vi "Parse Value.vi"(8 "error in (no error)":errorcluster, 11 "Alpaca CLI Parser in":refnum<class "JSON Parser.lvclass">) -> (0 "error out":errorcluster, 2 "Value":variant, 3 "Alpaca CLI Parser out":refnum<class "JSON Parser.lvclass">)   [LabVIEW 2013, in "JKI JSON Serialization.lvlib" / "JSON Parser.lvclass"]
uses:
  JSON Parser.lvclass
  Parser/Parser.lvclass/Parser.ctl
  JSON Lexer/JSON Token Type.ctl
  Parser/Lookahead.vi
  JSON Lexer/JSON Lexer.lvclass
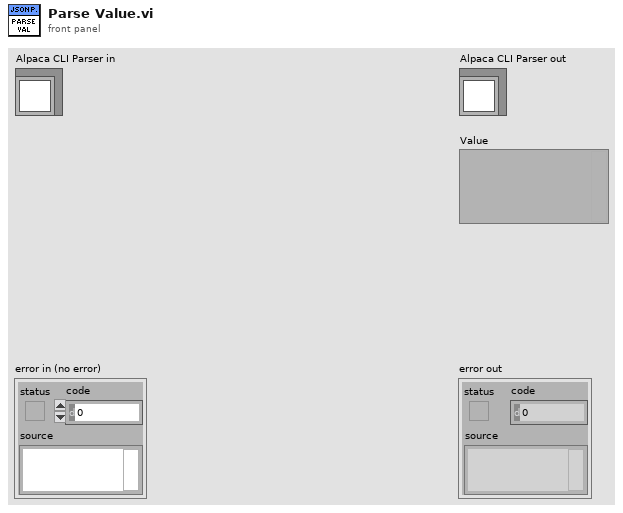
[diagram p1: front panel]
types:
  T1 = typedef "JKI JSON Serialization.lvlib/JSON Lexer.lvclass/JSON Token Type.ctl" = enum32{"unknown", "comma", "end-label", "begin-object", "end-object", "begin-array", "end-array", "quoted-string", "boolean", "exponential-number", "decimal-number", "integer-number", "special-number", "null", "symbol", "whitespace", "EOF"}
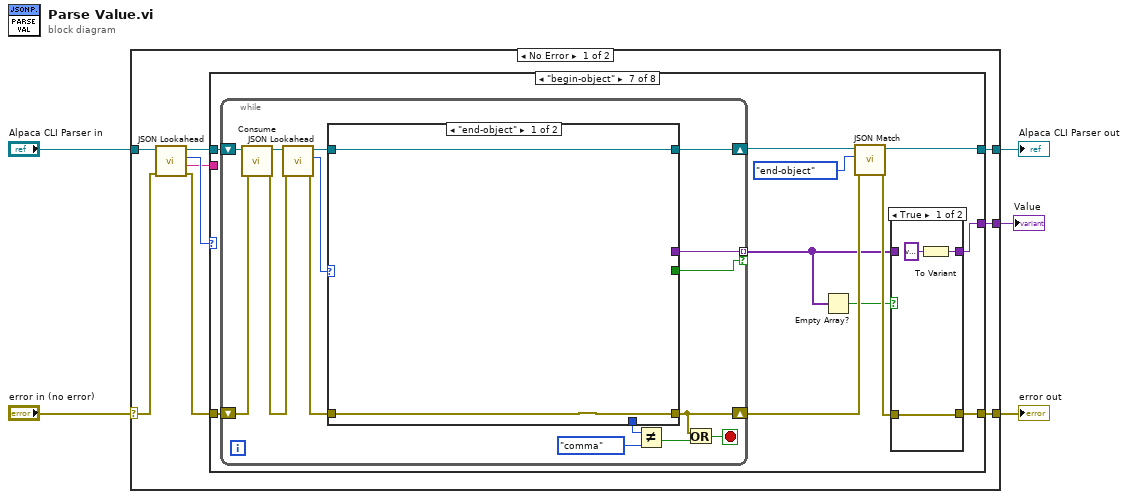
[diagram p0: block diagram]
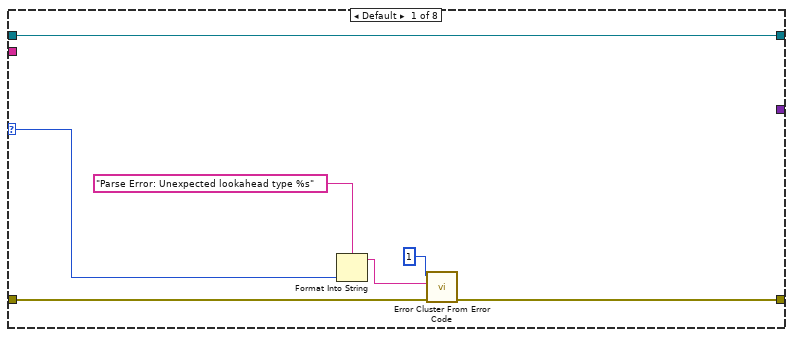
[diagram p2: hidden frame]
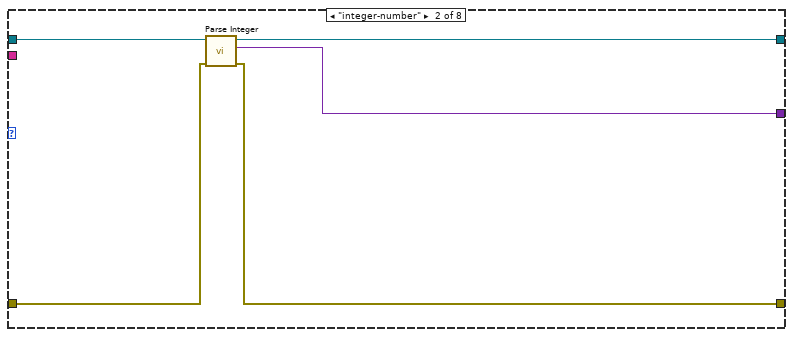
[diagram p3: hidden frame]
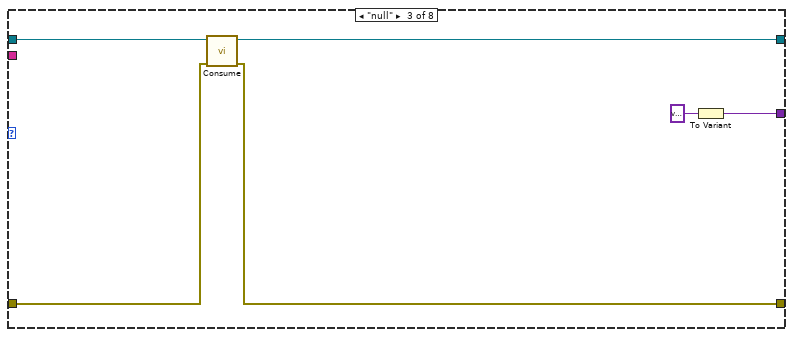
[diagram p4: hidden frame]
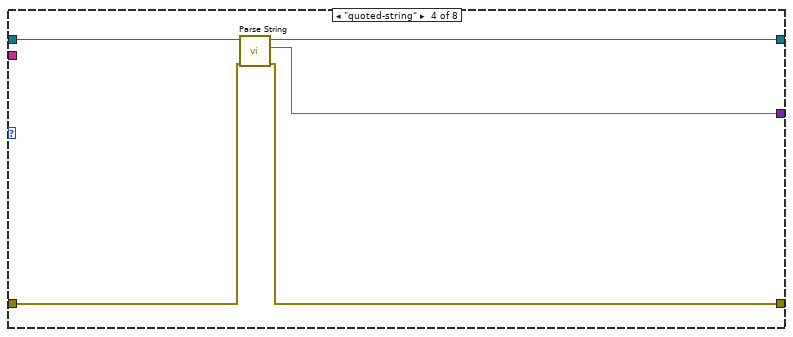
[diagram p5: hidden frame]
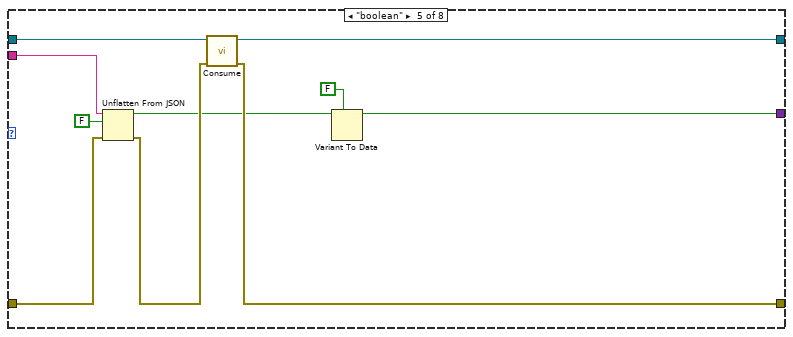
[diagram p6: hidden frame]
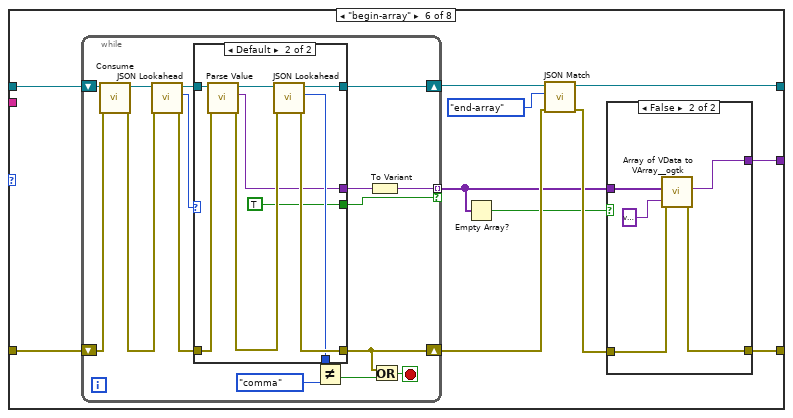
[diagram p7: hidden frame]
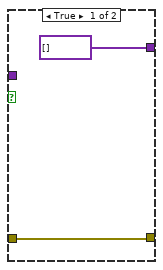
[diagram p8: hidden frame]
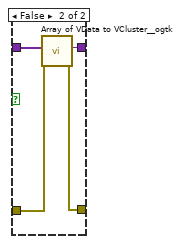
[diagram p10: hidden frame]
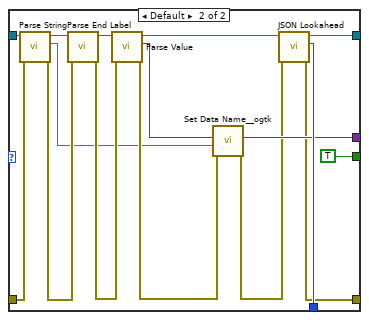
[diagram p11: hidden frame]
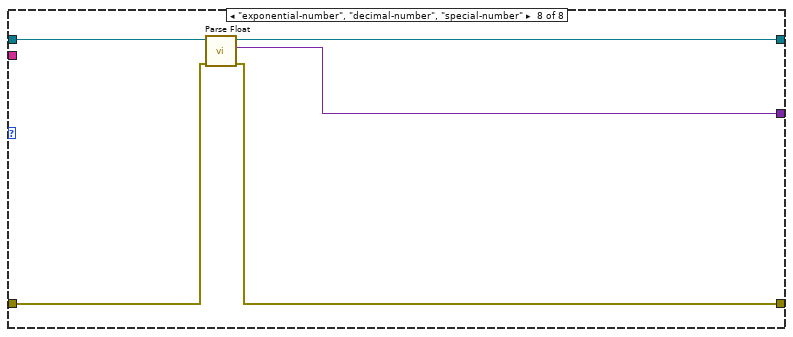
[diagram p12: hidden frame]
diagram:
  n1 = case shown="No Error" "error in (no error)" {
    selector: "error in (no error)" -> [w13 w151]
    tunnel: [w11 w151] -> w4
    tunnel: [w8 w150] -> w2
    tunnel: "Alpaca CLI Parser in" -> [w14 w150]
    tunnel: [w7 _] -> w1
    frame No Error {
      n2 = call "JSON Lookahead.vi"("error in (no error)"=w13, "Alpaca CLI Parser in"=w14) -> ("error out"=w9:errorcluster, "Lookahead Value"=w6:string, "Lookahead Type"=w10:T1, "Alpaca CLI Parser out"=w12:refnum<class "JSON Parser.lvclass">)  [unwired: 6 in]
      n3 = case shown="\"begin-object\"" w10 {
        selector: w10 -> [w17 _ _ _ _ _ _ _]
        tunnel: w12 -> [w15 w26 w32 w37 w47 w58 w104 w149]
        tunnel: [w15 w25 w31 w36 w46 w55 w101 w148] -> w8
        tunnel: [w21 w23 w29 w35 w45 w52 w97 w146] -> w11
        tunnel: w9 -> [w20 w24 w30 w33 w43 w57 w103 w147]
        tunnel: [_ w22 w27 w34 w39 w50 w98 w145] -> w7
        tunnel: w6 -> [_ _ _ _ w44 _ _ _]
        frame Default {
          n4 = Format Into String(format string="Parse Error: Unexpected lookahead type %s" ("error message (\"\")"), w17) -> (resulting string=w16:string)  [unwired: 2 in, 1 out]
          n5 = call <vilib>:"Error Cluster From Error Code.vi"("error in (no error)"=w20, "error message (\"\")"=w16, "error code (0)"=1) -> ("error out"=w21:errorcluster)  [unwired: 6 in]
        }
        frame "integer-number" {
          n6 = call-dynamic "Parse Integer.vi"("error in (no error)"=w24, "Alpaca CLI Parser in"=w26) -> ("error out"=w23:errorcluster, "Value"=w22:variant, "Alpaca CLI Parser out"=w25:refnum<class "JSON Parser.lvclass">)  [unwired: 7 in]
        }
        frame "null" {
          n7 = call-dynamic "Consume.vi"("error in (no error)"=w30, "Alpaca Parser in"=w32) -> ("error out"=w29:errorcluster, "Alpaca Parser out"=w31:refnum<class "JSON Parser.lvclass">)  [unwired: 8 in]
          n8 = To Variant(anything=variant ("Variant")) -> (Variant=w27:variant)
        }
        frame "quoted-string" {
          n9 = call "Parse String.vi"("error in (no error)"=w33, "JSON Parser in"=w37) -> ("error out"=w35:errorcluster, "Parsed String"=w34:string, "JSON Parser out"=w36:refnum<class "JSON Parser.lvclass">)  [unwired: 7 in]
        }
        frame "boolean" {
          n10 = Unflatten From JSON(JSON string=w44, type and defaults=FALSE, error in (no error)=w43) -> (value=w40:bool, error out=w42:errorcluster)  [unwired: 4 in]
          n11 = call-dynamic "Consume.vi"("error in (no error)"=w42, "Alpaca Parser in"=w47) -> ("error out"=w45:errorcluster, "Alpaca Parser out"=w46:refnum<class "JSON Parser.lvclass">)  [unwired: 8 in]
          n12 = Variant To Data(type=FALSE, Variant=w40) -> (data=w39:bool)  [unwired: 1 in, 1 out]
        }
        frame "begin-array" {
          n13 = while {
            shift-right: [w68] -> w54
            shift-left: w57 -> [w80]
            shift-right: [w77] -> w56
            shift-left: w58 -> [w81]
            tunnel: [w67] -> w49 mode=indexing if=w71
            stop <- w70 stop-if-true
            n14 = call-dynamic "Consume.vi"("error in (no error)"=w80, "Alpaca Parser in"=w81) -> ("error out"=w74:errorcluster, "Alpaca Parser out"=w76:refnum<class "JSON Parser.lvclass">)  [unwired: 8 in]
            n15 = call "JSON Lookahead.vi"("error in (no error)"=w74, "Alpaca CLI Parser in"=w76) -> ("error out"=w73:errorcluster, "Lookahead Type"=w72:T1, "Alpaca CLI Parser out"=w75:refnum<class "JSON Parser.lvclass">)  [unwired: 6 in, 1 out]
            n16 = case shown="Default" w72 {
              selector: w72 -> [w82 _]
              tunnel: [w83 w91] -> w68
              tunnel: [w82 w90] -> w78
              tunnel: [w84 w89] -> w77
              tunnel: [_ w88] -> w66
              tunnel: w75 -> [w84 w87]
              tunnel: w73 -> [w83 w86]
              tunnel: [_ TRUE] -> w71
              frame "end-array" {
              }
              frame Default {
                n17 = call-dynamic "Parse Value.vi"("error in (no error)"=w86, "Alpaca CLI Parser in"=w87) -> ("error out"=w92:errorcluster, "Value"=w88:variant, "Alpaca CLI Parser out"=w93:refnum<class "JSON Parser.lvclass">)  [unwired: 7 in]
                n18 = call "JSON Lookahead.vi"("error in (no error)"=w92, "Alpaca CLI Parser in"=w93) -> ("error out"=w91:errorcluster, "Lookahead Type"=w90:T1, "Alpaca CLI Parser out"=w89:refnum<class "JSON Parser.lvclass">)  [unwired: 6 in, 1 out]
              }
            }
            n19 = Not Equal?(x=w78, y=JSON_Token_Type."comma" ("Lookahead Type")) -> (x != y?=w69:bool)
            n20 = To Variant(anything=w66) -> (Variant=w67:variant)
            n21 = Or(x=w68, y=w69) -> (x .or. y?=w70:bool)
          }
          n22 = Empty Array?(array=w49) -> (empty?=w48:bool)
          n23 = call "JSON Match.vi"("error in (no error)"=w54, "JSON Token"=JSON_Token_Type."end-array" ("Lookahead Type"), "Alpaca CLI Parser in"=w56) -> ("error out"=w51:errorcluster, "Alpaca CLI Parser out"=w55:refnum<class "JSON Parser.lvclass">)  [unwired: 7 in]
          n24 = case shown="False" w48 {
            tunnel: [w59 w65] -> w52
            tunnel: w51 -> [w59 w64]
            tunnel: [variant[] [] w63] -> w50
            tunnel: w49 -> [_ w61]
            frame True {
            }
            frame False {
              n25 = call <userlib>:"Array of VData to VArray__ogtk.vi"("error in (no error)"=w64, "Element Type (when empty)"=variant, "1D Array of VData"=w61) -> ("error out"=w65:errorcluster, "VArray"=w63:variant)  [unwired: 7 in]
            }
          }
        }
        frame "begin-object" {
          n26 = while {
            shift-right: [w118] -> w100
            shift-left: w103 -> [w125]
            shift-right: [w122] -> w102
            shift-left: w104 -> [w126]
            tunnel: [w121] -> w94 mode=indexing if=w112
            stop <- w120 stop-if-true
            n27 = call-dynamic "Consume.vi"("error in (no error)"=w125, "Alpaca Parser in"=w126) -> ("error out"=w115:errorcluster, "Alpaca Parser out"=w117:refnum<class "JSON Parser.lvclass">)  [unwired: 8 in]
            n28 = call "JSON Lookahead.vi"("error in (no error)"=w115, "Alpaca CLI Parser in"=w117) -> ("error out"=w114:errorcluster, "Lookahead Type"=w113:T1, "Alpaca CLI Parser out"=w116:refnum<class "JSON Parser.lvclass">)  [unwired: 6 in, 1 out]
            n29 = case shown="\"end-object\"" w113 {
              tunnel: [_ w144] -> w123
              tunnel: [w128 w143] -> w122
              tunnel: [_ w142] -> w121
              tunnel: [w127 w141] -> w118
              tunnel: w116 -> [w128 w132]
              tunnel: w114 -> [w127 w131]
              tunnel: [_ TRUE] -> w112
              frame "end-object" {
              }
              frame Default {
                n30 = call "Parse String.vi"("error in (no error)"=w131, "JSON Parser in"=w132) -> ("error out"=w137:errorcluster, "Parsed String"=w133:string, "JSON Parser out"=w139:refnum<class "JSON Parser.lvclass">)  [unwired: 7 in]
                n31 = call-dynamic "Parse End Label.vi"("error in (no error)"=w137, "Alpaca CLI Parser in"=w139) -> ("error out"=w136:errorcluster, "Alpaca CLI Parser out"=w138:refnum<class "JSON Parser.lvclass">)  [unwired: 8 in]
                n32 = call-dynamic "Parse Value.vi"("error in (no error)"=w136, "Alpaca CLI Parser in"=w138) -> ("error out"=w135:errorcluster, "Value"=w129:variant, "Alpaca CLI Parser out"=w140:refnum<class "JSON Parser.lvclass">)  [unwired: 7 in]
                n33 = call <userlib>:"Set Data Name__ogtk.vi"("error in (no error)"=w135, "Data Name"=w133, "Data"=w129) -> ("error out"=w134:errorcluster, "Renamed Data"=w142:variant)  [unwired: 7 in]
                n34 = call "JSON Lookahead.vi"("error in (no error)"=w134, "Alpaca CLI Parser in"=w140) -> ("error out"=w141:errorcluster, "Lookahead Type"=w144:T1, "Alpaca CLI Parser out"=w143:refnum<class "JSON Parser.lvclass">)  [unwired: 6 in, 1 out]
              }
            }
            n35 = Not Equal?(x=w123, y=JSON_Token_Type."comma" ("Lookahead Type")) -> (x != y?=w119:bool)
            n36 = Or(x=w118, y=w119) -> (x .or. y?=w120:bool)
          }
          n37 = Empty Array?(array=w94) -> (empty?=w95:bool)
          n38 = call "JSON Match.vi"("error in (no error)"=w100, "JSON Token"=JSON_Token_Type."end-object" ("Lookahead Type"), "Alpaca CLI Parser in"=w102) -> ("error out"=w96:errorcluster, "Alpaca CLI Parser out"=w101:refnum<class "JSON Parser.lvclass">)  [unwired: 7 in]
          n39 = case shown="True" w95 {
            tunnel: [w105 w111] -> w98
            tunnel: [w107 w110] -> w97
            tunnel: w96 -> [w107 w109]
            tunnel: w94 -> [_ w108]
            frame True {
              n40 = To Variant(anything=variant ("Variant")) -> (Variant=w105:variant)
            }
            frame False {
              n41 = call <userlib>:"Array of VData to VCluster__ogtk.vi"("error in (no error)"=w109, "Array"=w108) -> ("error out"=w110:errorcluster, "VCluster"=w111:variant)  [unwired: 8 in]
            }
          }
        }
        frame "exponential-number", "decimal-number", "special-number" {
          n42 = call-dynamic "Parse Float.vi"("error in (no error)"=w147, "Alpaca CLI Parser in"=w149) -> ("error out"=w146:errorcluster, "Value"=w145:variant, "Alpaca CLI Parser out"=w148:refnum<class "JSON Parser.lvclass">)  [unwired: 7 in]
        }
      }
    }
    frame Error {
    }
  }
  "error out" <- w4
  "Alpaca CLI Parser out" <- w2
  "Value" <- w1
